vi "capt_data.vi"(7 "delay before read (ms)":u32, 8 "error in (no error)":errorcluster, 9 "sens_type_arry":T1 items=["SHTC3", "SHT3X", "D6T_1A", "HTS221", "AHT20", "ADT7410"], 10 "wr_buffr":string="\b", 11 "VISA Refnum in":refnum<visa-resource-name>) -> (0 "error out":errorcluster, 1 "bytes read":u32, 2 "Response":string, 3 "VISA Refnum out":refnum<visa-resource-name>)   [LabVIEW 2013]
uses:
  sens_type_arry_cntrl.ctl
  sens_type.ctl
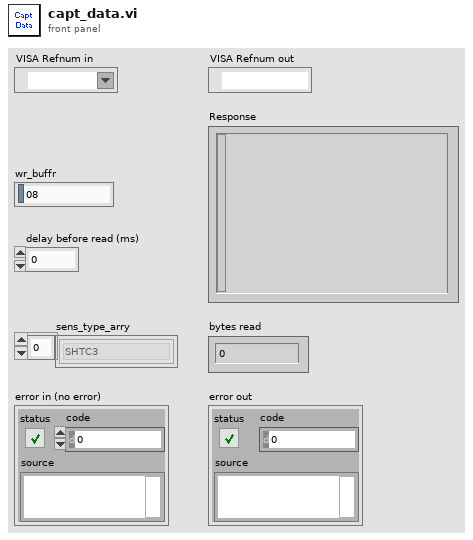
[diagram p1: front panel]
types:
  T1 = typedef "sens_type_arry_cntrl.ctl" = T2[]
  T2 = typedef "sens_type.ctl" = u8
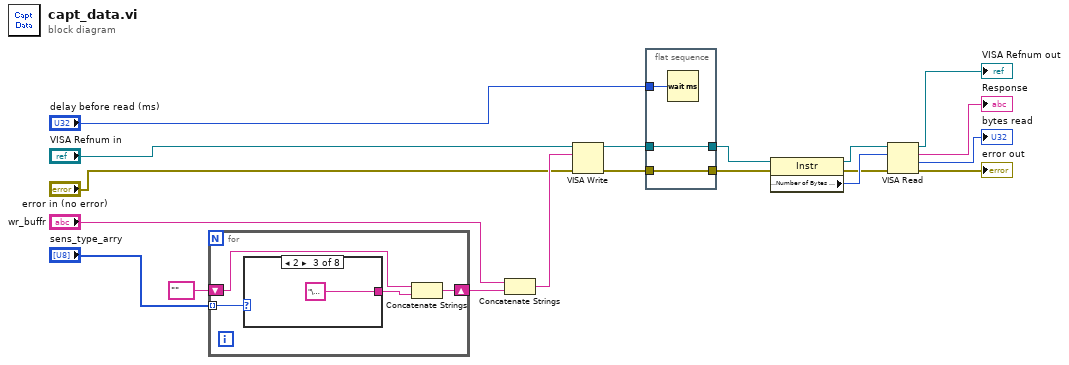
[diagram p0: block diagram]
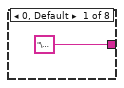
[diagram p2: hidden frame]
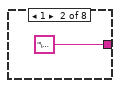
[diagram p3: hidden frame]
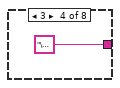
[diagram p4: hidden frame]
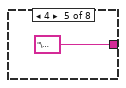
[diagram p5: hidden frame]
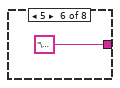
[diagram p6: hidden frame]
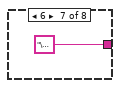
[diagram p7: hidden frame]
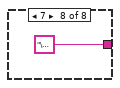
[diagram p8: hidden frame]
diagram:
  n1 = for {
    tunnel: "sens_type_arry" -> [w22] mode=indexing
    shift-right: [w21] -> w16
    shift-left: "" -> [w23]
    n2 = case shown="2" w22 {
      tunnel: ["\u0000" "\u0001" "\u0002" "\u0003" "\u0004" "\u0005" "\u0006" "\u0007"] -> w20
      frame 0, Default {
      }
      frame 1 {
      }
      frame 2 {
      }
      frame 3 {
      }
      frame 4 {
      }
      frame 5 {
      }
      frame 6 {
      }
      frame 7 {
      }
    }
    n3 = Concatenate Strings(w23, w20) -> (w21:string)
  }
  n4 = Concatenate Strings("wr_buffr", w16) -> (w19:string)
  n5 = VISA Write(VISA resource name="VISA Refnum in", write buffer=w19, error in (no error)="error in (no error)") -> (VISA resource name out=w3:refnum<visa-resource-name>, error out=w1:errorcluster)  [unwired: 1 out]
  n6 = flat-sequence {
    tunnel: w1 -> [w34]
    tunnel: [w34] -> w2
    tunnel: w3 -> [w33]
    tunnel: [w33] -> w4
    tunnel: "delay before read (ms)" -> [w32]
    frame #0 {
      n7 = Wait (ms)(milliseconds to wait=w32) -> ()  [unwired: 1 out]
    }
  }
  n8 = property class="Instr"(reference=w4, error in=w2) -> (reference out=w5:refnum<visa-resource-name>, error out=w6:errorcluster, "Serial Settings:Number of Bytes at Serial Port"=w8:u32)
  n9 = VISA Read(VISA resource name=w5, byte count=w8, error in (no error)=w6) -> (VISA resource name out=→"VISA Refnum out":refnum<visa-resource-name>, read buffer=→"Response":string, return count=→"bytes read":u32, error out=→"error out":errorcluster)
